vi "File.List All Files in a Directory Tree.vi"(8 "error in (no error)":errorcluster, 10 "Pattern":string, 11 "Folder":path) -> (0 "error out":errorcluster, 3 "Files":path[](array[path]))   [LabVIEW 2024, in "EQMF.lvlib" / "File Utils.lvlib"]
uses:
  File Utils.lvlib
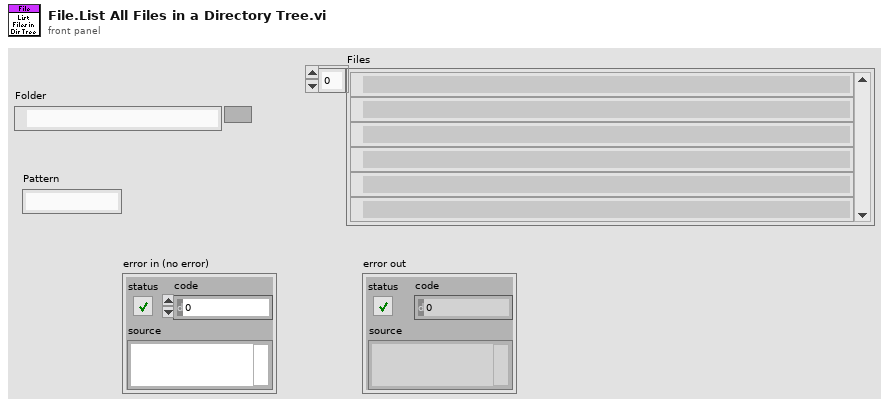
[diagram p1: front panel]
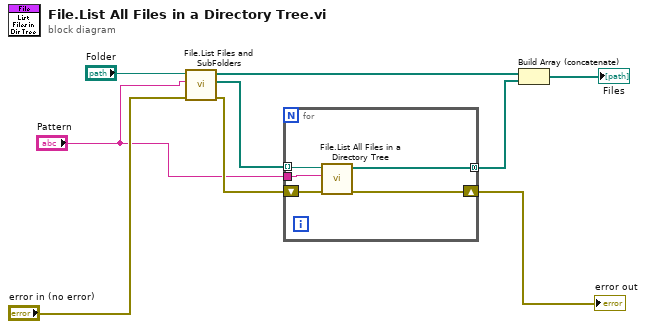
[diagram p0: block diagram]
diagram:
  n1 = call "File.List Files and SubFolders.vi"("error in"="error in (no error)", "Pattern"="Pattern", "Folder"="Folder") -> ("error out"=w3:errorcluster, "Folders"=w8:path[], "Files"=w7:path[])  [unwired: 6 in]
  n2 = for {
    tunnel: w8 -> [w14] mode=indexing
    tunnel: [w13] -> w6 mode=concatenating
    shift-right: [w11] -> w2
    shift-left: w3 -> [w12]
    tunnel: "Pattern" -> [w10]
    n3 = call "File.List All Files in a Directory Tree.vi"("error in (no error)"=w12, "Pattern"=w10, "Folder"=w14) -> ("error out"=w11:errorcluster, "Files"=w13:path[])  [unwired: 7 in]
  }
  "error out" <- w2
  n4 = Build Array (concatenate)(w7, w6) -> (→"Files":path[])
